vi "Import Export - Flatten to XML (CAR fix).vi"(8 "Error In":errorcluster, 10 "Export":T1 {"Tree"."Properties"."Type" items=["K_STRING", "K_BOOL", "K_I32", "K_U32", "K_DOUBLE", "K_U64", "K_VARIANT", "K_DEPENDENTFILE", "K_DEPENDENTNODE", "K_DATASOURCENODE", "K_U16", "K_DBLARR", "K_U32ARR", "K_I32ARR", "K_STRINGARR", "K_DICTIONARY", "K_DICTIONARYARR"]}) -> (0 "Error Out":errorcluster, 2 "XML String Out":string)   [LabVIEW 2017, in "Scan Engine Custom Device.lvlib"]
doc: "Flattern exported data to XML. It contains a workaround the CAR #198717."
uses:
  Scan Engine Custom Device.lvlib
  <vilib>/NI/NI VeriStand Advanced SysDef API/_Types/SysDef.Export.ctl
  <vilib>/NI/NI VeriStand Advanced SysDef API/_Types/TreeItem.ctl
  <vilib>/NI/NI VeriStand Advanced SysDef API/_Types/TreeItem.Info.ctl
  <vilib>/NI Veristand/Custom Device API/Custom Device Channel.ctl
  <vilib>/NI Veristand/Custom Device API/Custom Device Channel Type.ctl
  <vilib>/NI Veristand/Custom Device API/Custom Device Waveform.ctl
  <vilib>/NI Veristand/Custom Device API/Custom Device Waveform DataType.ctl
  <vilib>/NI/NI VeriStand Advanced SysDef API/_Types/TreeItem.Property.ctl
  <vilib>/NI/NI VeriStand Advanced SysDef API/SysDef API/Advanced System Definition.lvlib
  <vilib>/NI Veristand/Custom Device API/Custom Device API.lvlib
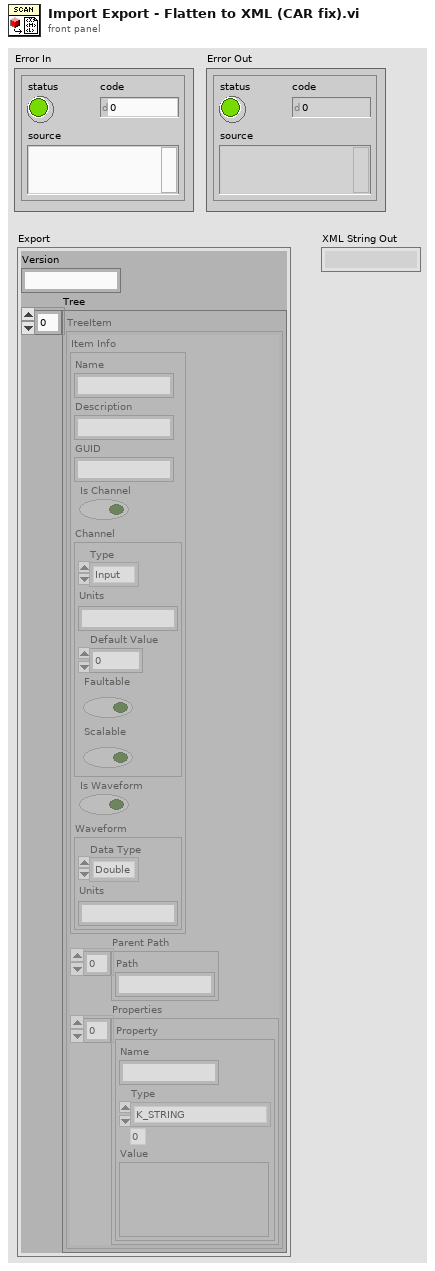
[diagram p1: front panel]
types:
  T1 = typedef "Advanced System Definition.lvlib/SysDef.Export.ctl" = cluster{"Version":string, "Tree":T2[]}
  T2 = typedef "Advanced System Definition.lvlib/TreeItem.ctl" = cluster{"Item Info":T3, "Parent Path":string[], "Properties":T8[]}
  T3 = typedef "Advanced System Definition.lvlib/TreeItem.Info.ctl" = cluster{"Name":string, "Description":string, "GUID":string, "Is Channel":bool, "Channel":T4, "Is Waveform":bool, "Waveform":T6}
  T4 = typedef "Custom Device API.lvlib/Custom Device Channel.ctl" = cluster{"Type":T5, "Units":string, "Default Value":dbl, "Faultable":bool, "Scalable":bool}
  T5 = typedef "Custom Device API.lvlib/Custom Device Channel Type.ctl" = enum16{"Input", "Output"}
  T6 = typedef "Custom Device API.lvlib/Custom Device Waveform.ctl" = cluster{"Data Type":T7, "Units":string}
  T7 = typedef "Custom Device API.lvlib/Custom Device Waveform DataType.ctl" = enum16{"Double", "Complex Double"}
  T8 = typedef "Advanced System Definition.lvlib/TreeItem.Property.ctl" = cluster{"Name":string, "Type":i32, "Value":variant}
  T9 = cluster{"type string":i16[], "data string":string}
  T10 = cluster{"Name":string, "Type":i32, cluster{"type string":i16[], "data string":string}}
  T11 = cluster{"Item Info":T3, "Parent Path":string[], cluster{"Name":string, "Type":i32, cluster{"type string":i16[], "data string":string}}[]}
  T12 = cluster{"Version":string, cluster{"Item Info":T3, "Parent Path":string[], cluster{"Name":string, "Type":i32, cluster{"type string":i16[], "data string":string}}[]}[]}
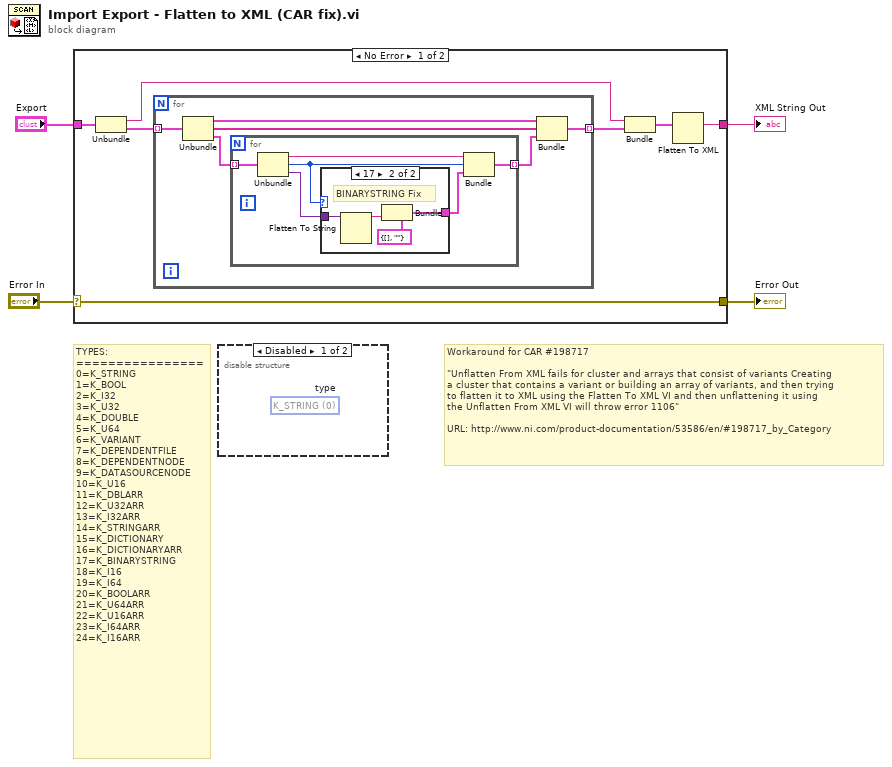
[diagram p0: block diagram]
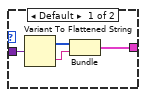
[diagram p2: hidden frame]
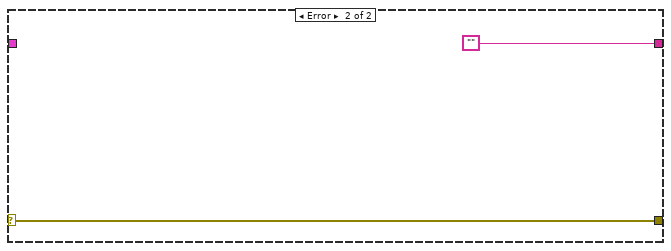
[diagram p3: hidden frame]
diagram:
  # "Workaround for CAR #198717\n\n\"Unflatten From XML fails for cluster and arrays that consist of variants Creating\na cluster that contains a variant or building an array of variants, and then trying\nto flatten it to XML using the Flatten To XML VI and then unflattening it using\nthe Unflatten From XML VI will throw error 1106\"\n\nURL: http://www.ni.com/product-documentation/53586/en/#198717_by_Category"
  # "TYPES:\n================\n0=K_STRING\n1=K_BOOL\n2=K_I32\n3=K_U32\n4=K_DOUBLE\n5=K_U64\n6=K_VARIANT\n7=K_DEPENDENTFILE\n8=K_DEPENDENTNODE\n9=K_DATASOURCENODE\n10=K_U16\n11=K_DBLARR\n12=K_U32ARR\n13=K_I32ARR\n14=K_STRINGARR\n15=K_DICTIONARY\n16=K_DICTIONARYARR\n17=K_BINARYSTRING\n18=K_I16\n19=K_I64\n20=K_BOOLARR\n21=K_U64ARR\n22=K_U16ARR\n23=K_I64ARR\n24=K_I16ARR"
  n1 = case shown="No Error" "Error In" {
    selector: "Error In" -> [w10 w33]
    tunnel: [w11 ""] -> w4
    tunnel: "Export" -> [w9 _]
    tunnel: [w10 w33] -> w1
    frame No Error {
      n2 = Unbundle(w9) -> ("Version"=w5:string, "Tree"=w8:T2[])
      n3 = for {
        tunnel: w8 -> [w17] mode=indexing
        tunnel: [w14] -> w6 mode=indexing
        n4 = Unbundle(w17) -> ("Item Info"=w16:T3, "Parent Path"=w15:string[], "Properties"=w13:T8[])
        n5 = for {
          tunnel: w13 -> [w23] mode=indexing
          tunnel: [w20] -> w12 mode=indexing
          n6 = Unbundle(w23) -> ("Name"=w19:string, "Type"=w18:i32, "Value"=w22:variant)
          n7 = case shown="17" w18 {
            tunnel: w22 -> [w27 w29]
            tunnel: [w25 w31] -> w21
            frame Default {
              n8 = Variant To Flattened String(Variant=w27) -> (data string=w26:string, 1:w24:i16[])
              n9 = Bundle("type string"=w24, "data string"=w26) -> (w25:T9)  [unwired: 1 in]
            }
            frame 17 {
              # "BINARYSTRING Fix"
              n10 = Flatten To String(anything=w29) -> (data string=w28:string)  [unwired: 3 in, 2 out]
              n11 = Bundle(cluster=T9 {"type string"=[], "data string"=""}, "data string"=w28) -> (w31:T9)  [unwired: 1 in]
            }
          }
          n12 = Bundle("Name"=w19, "Type"=w18, w21) -> (w20:T10)  [unwired: 1 in]
        }
        n13 = Bundle("Item Info"=w16, "Parent Path"=w15, w12) -> (w14:T11)  [unwired: 1 in]
      }
      n14 = Bundle("Version"=w5, w6) -> (w7:T12)  [unwired: 1 in]
      n15 = Flatten To XML(anything=w7) -> (xml string=w11:string)
    }
    frame Error {
    }
  }
  "XML String Out" <- w4
  "Error Out" <- w1
  n16 = disable-structure shown="Disabled" {
    frame Disabled {
      (unwired) 0 items=["K_STRING", "K_BOOL", "K_I32", "K_U32", "K_DOUBLE", "K_U64", "K_VARIANT", "K_DEPENDENTFILE", "K_DEPENDENTNODE", "K_DATASOURCENODE", "K_U16", "K_DBLARR", "K_U32ARR", "K_I32ARR", "K_STRINGARR", "K_DICTIONARY", "K_DICTIONARYARR", "K_BINARYSTRING", "K_I16", "K_I64", "K_BOOLARR", "K_U64ARR", "K_U16ARR", "K_I64ARR", "K_I16ARR"]  # type
    }
    frame Enabled {
    }
  }
